vi "EvaluatePass.vi"(7 "Gap Coord":dbl[](array[numeric]), 8 "error in (no error)":errorcluster, 9 "Game":refnum<class "Game.lvclass">, 10 "Point":dbl[](array[numeric]), 11 "object in":refnum<class "Utilities.lvclass">) -> (0 "error out":errorcluster, 2 "evaluation":dbl, 3 "object out":refnum<class "Utilities.lvclass">)   [LabVIEW 2023, in "Utilities.lvclass"]
uses:
  Utilities.lvclass
  Game_class/Game.lvclass
  Game_class/Game.lvclass/Game.ctl
  Parameters_class/Parameters.lvclass/Parameters.ctl
  Object_class/Object.lvclass/Object.ctl
  Game_class/Read Parameters.lvclass.vi
  Game_class/Read NewParameters.vi
  Game_class/Read BallRef.vi
  Object_class/Read position(x,y).vi
  Parameters_class/Read AttakingOurselves.vi
  Ball_class/Ball.lvclass
  Parameters_class/Parameters.lvclass
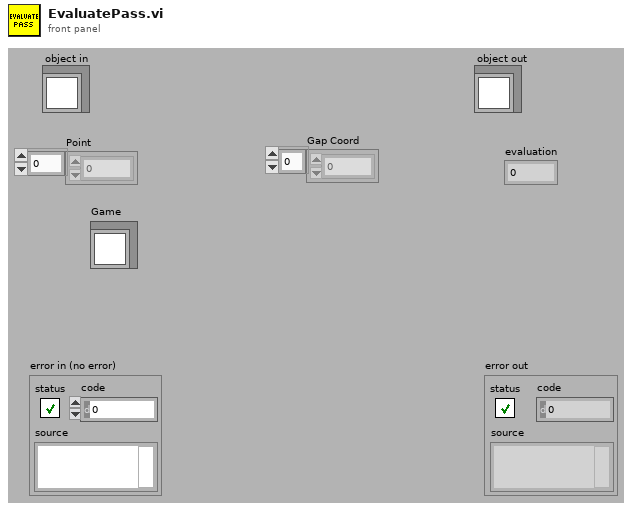
[diagram p1: front panel]
types:
  T1 = typedef "NewParameters.ctl" = cluster{"PenaltyDistance":dbl, "DistanceAttackerToBackBall":dbl, "Division":enum16{"Div B", "Div A"}, "DistanceToAvoidyEnemyRobot":dbl, "BallPlacementDistance":dbl, "DisatanceBehindBallToStealBall":dbl, "MaxDistanceToPositionKickoff":dbl, "BlockEnemyTarget":bool, "MaxStopVAng":dbl, "DistanceMarkerToEnemy":dbl, "IgnoreDribblerContact":bool, "DistanceToBeginEnemyPosession":dbl, "GoToBallWhenEnemyNotMoving":bool, "EnemyDistanceToReduceVelocity":dbl, "TurnOnEnemyDistanceToReduceVelocity":bool, "EnemyDistanceToShootOutBall":dbl, "DefenseKickBall":bool, "MoreKickToGoal? (0-0.3)":dbl, "ChipKickInEnemyField":bool, "ShootOutRobotId":dbl, "FieldLenghtDenominatorInShootOut":dbl, "AdjustPositionInBallPlacement":bool, "PowerGodPass":dbl, "VelocityAbortEnemyPos":dbl, "MaxDistToBeginPass":dbl, "MinDistToBeginPass":dbl, "VelocityInDirects":dbl, "BadDribblerIDs":i32[], "NewKickToDistanceAroundBall":dbl, "PowerAvoidColisionMarker":dbl, "DistanceToAvoidColisionMarker":dbl, "AvoidBallKick":dbl, "DistanceTryKick":dbl, "SuicideKickDIstance":dbl, "AdjustFirstKickDistance":dbl, "AvoidAimLessKick":dbl, "DistanceToAvoidyEnemyShootRobot ":dbl, "NumberOfMarkers":dbl, "PotField":bool, "PIDLateral":bool, "MinDistanceFirstKickX":dbl, "MinDistanceFirstKickY":dbl, "FractionOfDistToTouchGround\nAfterChipKick":dbl, "FractionOfKickxWhen\nComposedWithKickz":dbl, "Style":T2, "MoveInTurnState":bool, "DistFromEnemyToConsider\nMoveInTurnState":dbl, "CascadePID":bool, "TurnAroundParameters":cluster{"Radius":dbl, "Multiplier":dbl, "ChordAngle":dbl}, "SafeDriveVel":dbl, "DistanceToGoToBackBall":dbl, "minDistanceToNotFinishEnemyPossession":dbl, "OneTouchShot":cluster{"angleFactor":dbl, "maxAngle":dbl, "Attack":bool, "Defense":bool}, "OpenAngleToGoal":cluster{"minAngle":dbl, "maxAngle":dbl, "minEvaluation":dbl}, "ShotInterception":cluster{"shotSpeed":dbl, "minEnemySpeed":dbl, "maxEnemySpeed":dbl, "minEvaluation":dbl}, "AllyTeamArray":T3[], "maxDefendersNumber":i32, "Zone":cluster{"GuardPositionArray":dbl[][], "ZoneMidField":dbl[], "CenterForwardWidth":dbl}, "MinEvaluationToShoot":dbl, "PassInterception":cluster{"maxPassSpeed":dbl, "minPassSpeed":dbl, "minEnemySpeed":dbl, "chipPassDistance":dbl, "chipPassEvaluation":dbl, "minEvaluation":dbl, "maxEnemySpeed":dbl}, "PassDistance":cluster{"maxDistance":dbl, "minDistance":dbl}}
  T2 = typedef "Style.ctl" = enum16{"Insanity", "Offensive", "Defensive"}
  T3 = typedef "AllyTeam.ctl" = enum16{"Keeper", "Defender", "Attacker"}
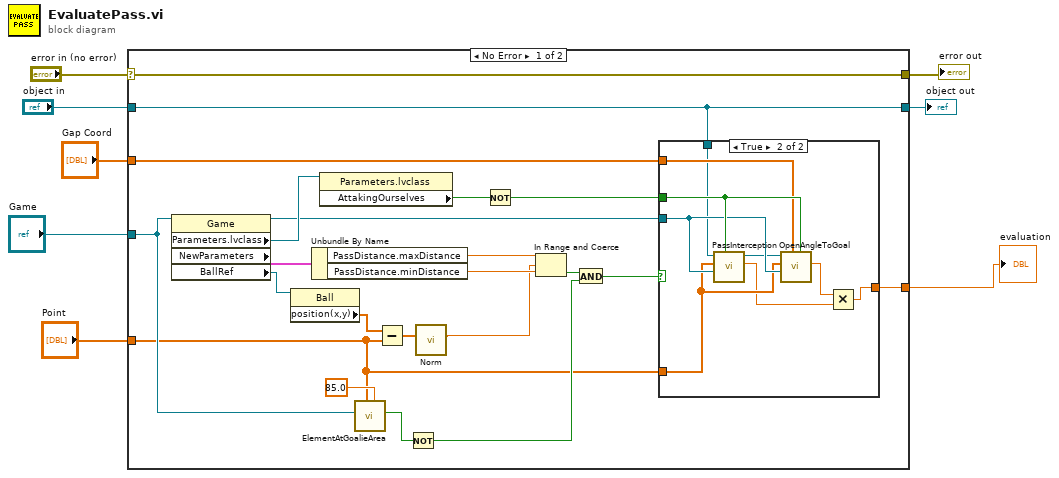
[diagram p0: block diagram]
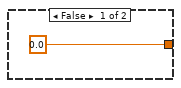
[diagram p2: hidden frame]
diagram:
  n1 = case shown="No Error" "error in (no error)" {
    selector: "error in (no error)" -> [w30 w42]
    tunnel: [w30 w42] -> w7
    tunnel: [w10 w41] -> w5
    tunnel: "object in" -> [w10 w41]
    tunnel: "Game" -> [w22 _]
    tunnel: "Point" -> [w12 _]
    tunnel: [w17 _] -> w2
    tunnel: "Gap Coord" -> [w13 _]
    frame No Error {
      n2 = property class="Game"(reference=w22) -> (reference out=w11:refnum<class "Game.lvclass">, "Parameters.lvclass"=w16:refnum<class "Parameters.lvclass">, "NewParameters"=w29:T1, "BallRef"=w28:refnum<class "Ball.lvclass">)  [unwired: 1 in, 1 out]
      n3 = property class="Ball"(reference=w28) -> ("position(x,y)"=w27:dbl[])  [unwired: 1 in, 2 out]
      n4 = Unbundle By Name(w29) -> ("PassDistance.maxDistance"=w26:dbl, "PassDistance.minDistance"=w25:dbl)
      n5 = property class="Parameters.lvclass"(reference=w16) -> ("AttakingOurselves"=w15:bool)  [unwired: 1 in, 2 out]
      n6 = call "ElementAtGoalieArea.vi"("ElementRadius"=85.0, "Elemento pos."=w12, "Game"=w22) -> ("Element at any goalkeeper area ?"=w9:bool)  [unwired: 4 in, 4 out]
      n7 = Subtract(x=w27, y=w12) -> (x-y=w24:dbl[])
      n8 = Not(x=w9) -> (.not. x?=w19:bool)
      n9 = call "Norm.vi"("2D vector"=w24) -> ("Modulo"=w23:dbl)  [unwired: 8 in, 2 out]
      n10 = Not(x=w15) -> (.not. x?=w14:bool)
      n11 = In Range and Coerce(upper limit=w26, x=w23, lower limit=w25) -> (In Range?=w20:bool)  [unwired: 1 out]
      n12 = And(x=w20, y=w19) -> (x .and. y?=w18:bool)
      n13 = case shown="True" w18 {
        tunnel: [0.0 ("evaluation") w34] -> w17
        tunnel: w14 -> [_ w40]
        tunnel: w13 -> [_ w39]
        tunnel: w12 -> [_ w37]
        tunnel: w11 -> [_ w38]
        tunnel: w10 -> [_ w32]
        frame False {
        }
        frame True {
          n14 = call "PassInterception.vi"("Ally?"=w40, "Game"=w38, "Point"=w37, "object in"=w32) -> ("Evaluation"=w35:dbl, "object out"=w33:refnum<class "Utilities.lvclass">)  [unwired: 5 in, 1 out]
          n15 = call "OpenAngleToGoal.vi"("Ally?"=w40, "Gap Coord"=w39, "Game"=w38, "Point"=w37, "object in"=w33) -> ("Evaluation"=w36:dbl)  [unwired: 4 in, 2 out]
          n16 = Multiply(x=w36, y=w35) -> (x*y=w34:dbl)
        }
      }
    }
    frame Error {
    }
  }
  "error out" <- w7
  "object out" <- w5
  "evaluation" <- w2
